vi "LoadRefs.vi"(0 "Number of axes":i32=8, 1 "Number of refs":i32=4, 3 "error in":errorcluster) -> (8 "Références à enregistrer":dbl[][](array[numeric]), 10 "error out":errorcluster)   [LabVIEW 2013]
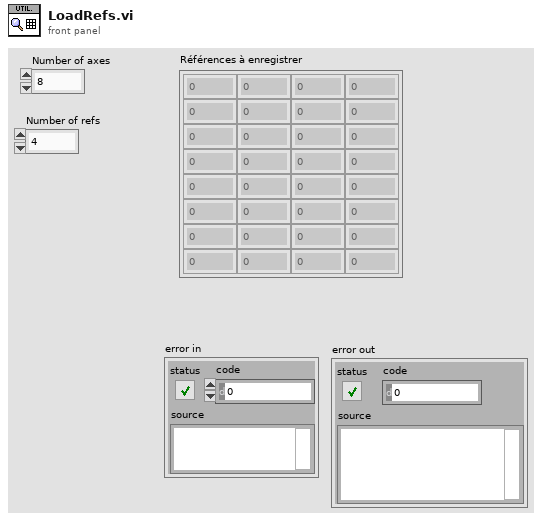
[diagram p1: front panel]
types:
  T1 = enum16{"open", "replace", "create", "open or create", "replace or create", "replace or create with confirmation"}
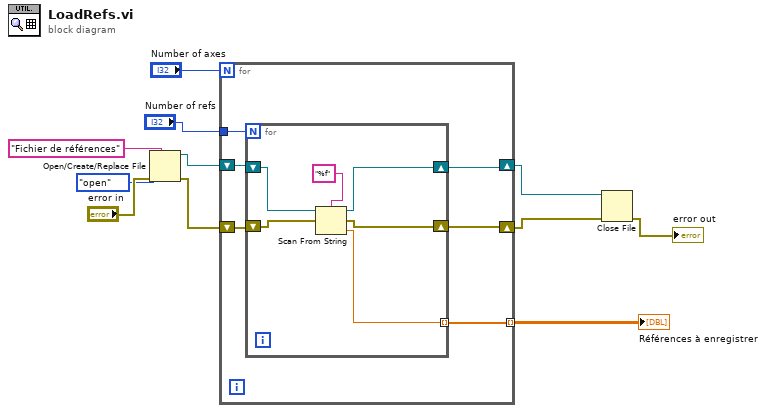
[diagram p0: block diagram]
diagram:
  n1 = Open/Create/Replace File(error in="error in", prompt="Fichier de références", operation (0:open)=T1."open") -> (refnum out=w5:refnum<file>, error out=w7:errorcluster)  [unwired: 3 in, 1 out]
  n2 = for {
    N: "Number of axes" -> [_]
    shift-right: [w13] -> w3
    shift-left: w7 -> [w17]
    tunnel: [w16] -> w6 mode=indexing
    shift-right: [w14] -> w4
    shift-left: w5 -> [w15]
    tunnel: "Number of refs" -> [w12]
    n3 = for {
      N: w12 -> [_]
      shift-right: [w21] -> w13
      shift-left: w17 -> [w22]
      shift-right: [w18] -> w14
      shift-left: w15 -> [w19]
      tunnel: [w20] -> w16 mode=indexing
      n4 = Scan From String("%f" ("format string"), w19, w22) -> (w18:refnum<file>, w21:errorcluster, output 1=w20:dbl)  [unwired: 1 in]
    }
  }
  "Références à enregistrer" <- w6
  n5 = Close File(refnum=w4, error in=w3) -> (error out=→"error out":errorcluster)  [unwired: 1 out]
